vi "get_object.vi"(0 "HGF_FGV_Index":refnum<class "HGF_FGV_Index.lvclass">, 5 "error in (no error)":errorcluster) -> (14 "dup HGF_FGV_Index":refnum<class "HGF_FGV_Index.lvclass">, 16 "object":refnum<class>, 19 "error out":errorcluster)   [LabVIEW 2012, in "HGF_FGV.lvlib" / "HGF_FGV_Index.lvclass"]
doc: "Returns the indexed object."
uses:
  HGF_FGV_Index.lvclass
  HGF_FGV_Index.lvclass/HGF_FGV_Index.ctl
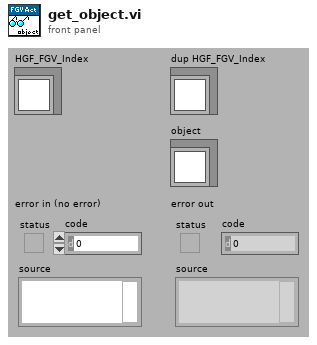
[diagram p1: front panel]
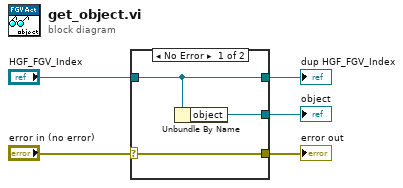
[diagram p0: block diagram]
diagram:
  n1 = case shown="No Error" "error in (no error)" {
    selector: "error in (no error)" -> [w8 w9]
    tunnel: [w8 w9] -> w4
    tunnel: [w7 w10] -> w2
    tunnel: "HGF_FGV_Index" -> [w7 w10]
    tunnel: [w6 _] -> w1
    frame No Error {
      n2 = Unbundle By Name(w7) -> ("object"=w6:refnum<class>)
    }
    frame Error {
    }
  }
  "error out" <- w4
  "dup HGF_FGV_Index" <- w2
  "object" <- w1
